vi "MoveSinglePIMotor.vi"(0 "System no.":i32=1 min=1 step=1, 1 "Axes to move":string[](array[string]), 2 "Move":dbl[](array[numeric]) format="%.6f", 3 "SafeMax":dbl[](array[numeric]) format="%.6f", 4 "SafeMin":dbl[](array[numeric]) format="%.6f", 5 "error in":errorcluster, 6 "Define home":bool, 7 "Move relative (-)":bool, 8 "Go home":bool, 9 "Move relative (+)":bool, 11 "Move absolute":bool, 12 "Stop refnum":refnum<vi>) -> (15 "Position":dbl[](array[numeric]) format="%.6f", 19 "error out":errorcluster)   [LabVIEW 2013]
doc: "This VI is runs in a loop until the stop button is pressed, the stop reference is TRUE or an error occures. It lets the operator set the velocity, move the connected axes to relative, absolute or to the home position, and reads the current position continuosly. The diagram shows how to combine the driver and support VIs for these tasks. Use the Help?Show Context Help menu sequence in the LabVIEW environment to display the Context Help window with the VI and control/indicator descriptions.\nRun \" XXXX_Configuration_Setup.vi\" (with XXXX being the PI product number of your system) prior to running this VI. \n\nValid for: C-843, C-843.PM, C-865, C-866, Mercury"
uses:
  C:/Users/Public/PI/GCSMergedLabVIEW/Low Level/General command.llb/Global2 (Array).vi
panel:
  in  "Clear":bool
  in  "stop":bool
  out "Conn. Axes":string[](array[string])
  # "Command move:"
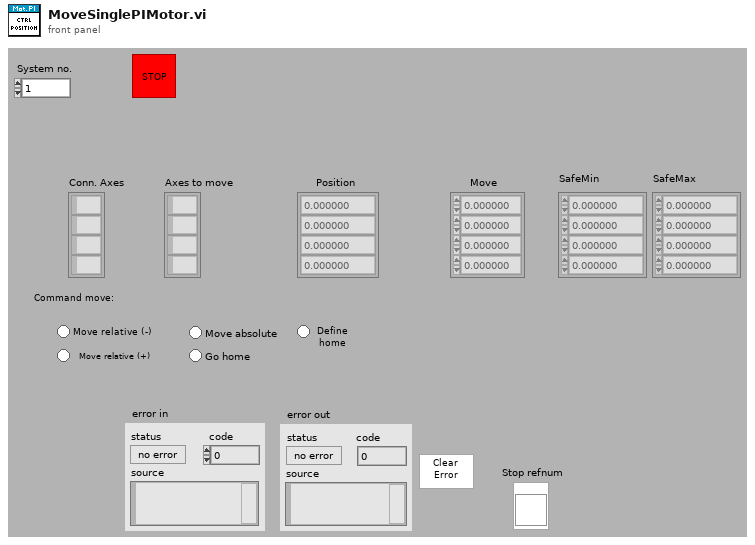
[diagram p1: front panel]
types:
  T1 = typedef "Controller names.ctl" = enum16{"None", "Analog", "C-702", "C-413", "C-843", "C-843.PM", "C-844", "C-848", "C-865", "C-866", "C-867", "C-877", "C-880", "C-884", "C-885", "C-891", "E-516", "E-517", "E-518", "E-709", "E-710", "E-712", "E-725", "E-727", "E-753", "E-754", "E-755", "E-761", "E-816", "E-861", "E-870", "E-871", "E-873", "F-206", "HydraPollux", "M-840", "M-850", "M-8X0", "Mercury", "Mercury_GCS"}
  T2 = cluster{"Conn. axes":string[], "Controller name":T1}[]
  T3 = cluster{"Conn. axes":string[], "Controller name":T1}
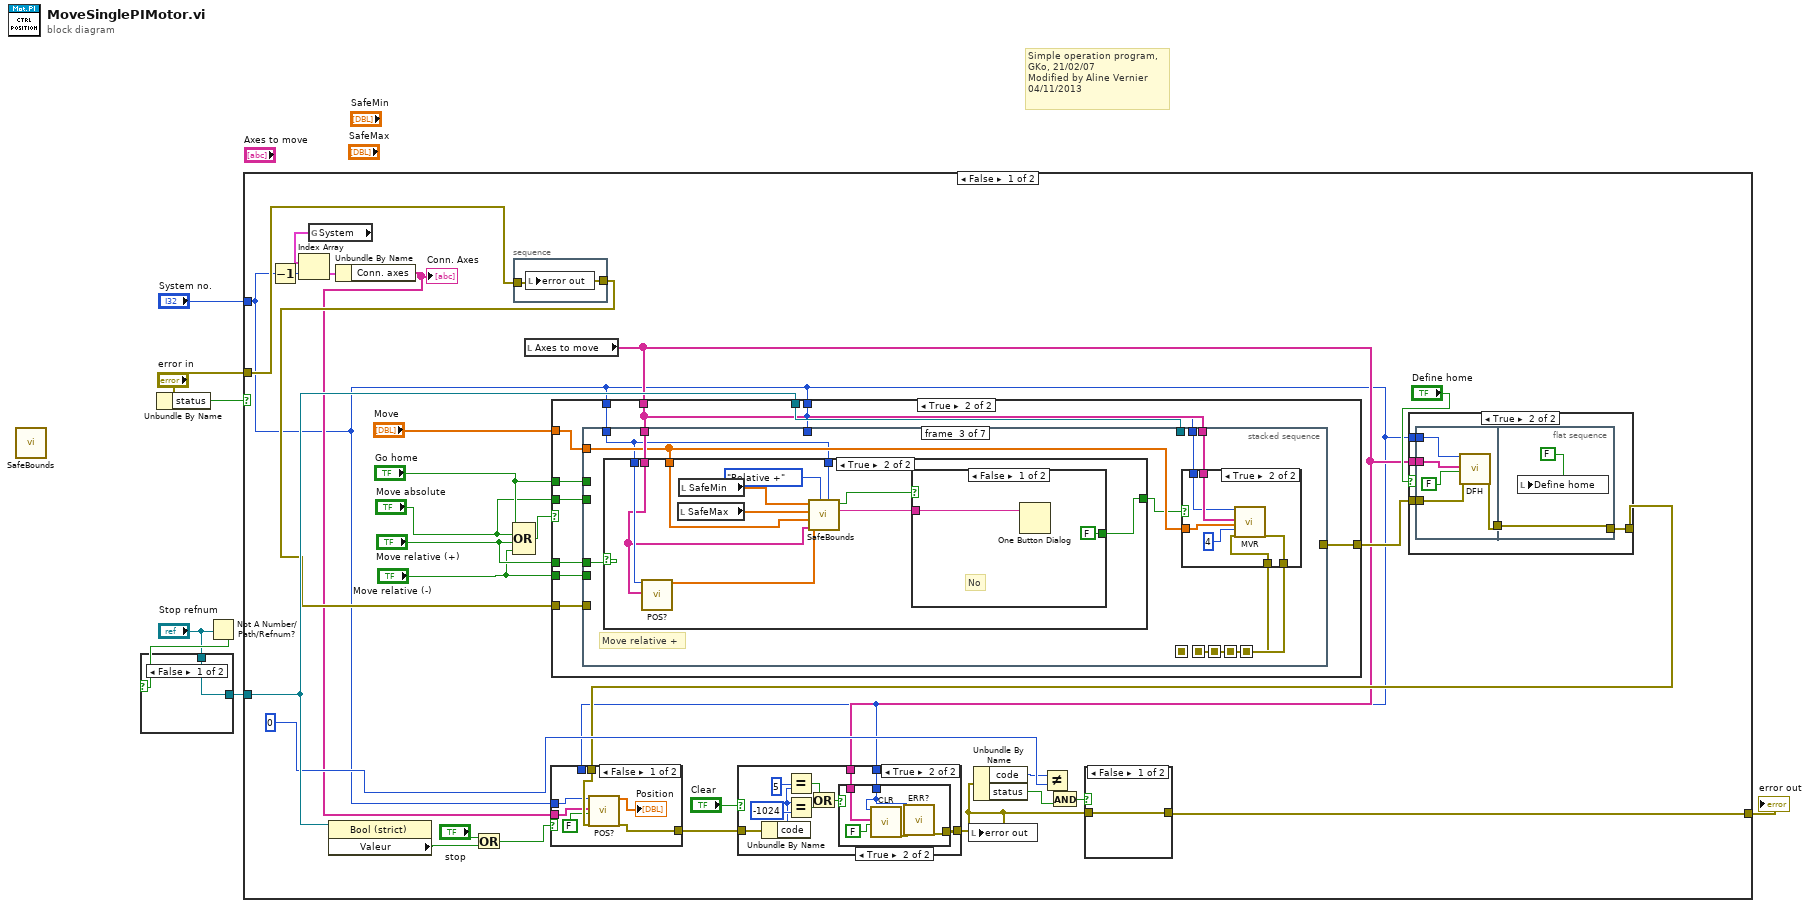
[diagram p0: block diagram]
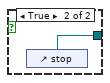
[diagram p2: hidden frame]
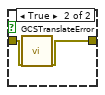
[diagram p3: hidden frame]
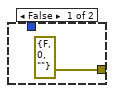
[diagram p5: hidden frame]
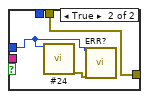
[diagram p6: hidden frame]
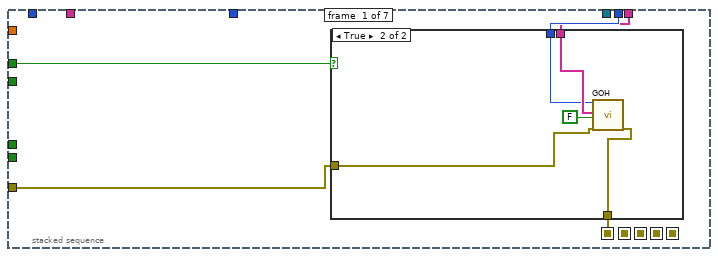
[diagram p8: hidden frame]
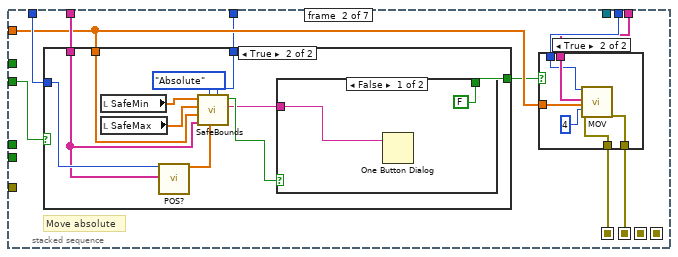
[diagram p10: hidden frame]
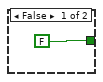
[diagram p11: hidden frame]
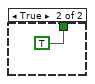
[diagram p12: hidden frame]
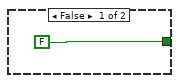
[diagram p14: hidden frame]
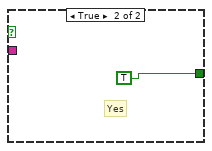
[diagram p15: hidden frame]
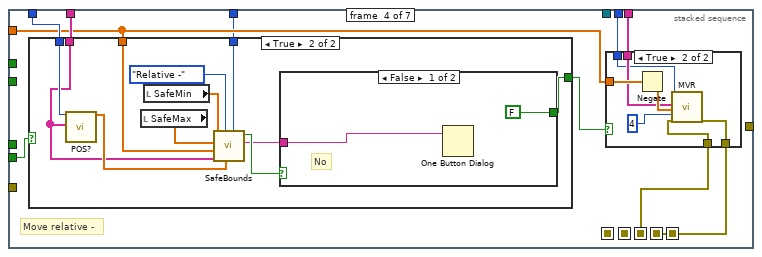
[diagram p17: hidden frame]
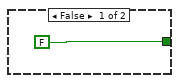
[diagram p18: hidden frame]
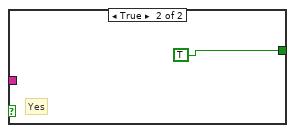
[diagram p19: hidden frame]
diagram:
  # "Simple operation program,\nGKo, 21/02/07\nModified by Aline Vernier\n04/11/2013"
  n1 = call "SafeBounds.vi"() -> ()  [unwired: 9 in, 3 out]
  n2 = Unbundle By Name("error in") -> ("status"=w6:bool)
  n3 = Not A Number/Path/Refnum?(number/path/refnum="Stop refnum") -> (NaN/Path/Refnum?=w3:bool)
  n4 = case shown="False" w3 {
    tunnel: [w8 w9] -> w2
    tunnel: "Stop refnum" -> [w8 _]
    frame False {
    }
    frame True {
      n5 = control-ref of="stop"() -> (w9:refnum<vi>)
    }
  }
  n6 = case shown="False" w6 {
    tunnel: [w39 w220] -> w5
    tunnel: "error in" -> [w38 w220]
    tunnel: "System no." -> [w10 _]
    tunnel: w2 -> [w37 _]
    frame False {
      n7 = Decrement(x=w10) -> (x-1=w35:i32)
      n8 = global read "Global2 (Array).vi" "System"() -> (w34:T2)
      n9 = Index Array(array=w34, index=w35) -> (element=w33:T3)
      n10 = property class="Bool (strict)"(reference=w37) -> ("Valeur"=w27:bool)  [unwired: 1 in, 2 out]
      n11 = Unbundle By Name(w33) -> ("Conn. axes"=w12:string[])
      "Conn. Axes" <- w12
      n12 = Or(x="stop", y=w27) -> (x .or. y?=w13:bool)
      n13 = Compound Arithmetic op=OR("Go home", "Move absolute", "Move relative (+)", "Move relative (-)") -> (w15:bool)
      n14 = stacked-sequence {
        tunnel: w38 -> [w219]
        tunnel: [w219] -> w32
        frame #0 {
          n15 = local write "error out"(w219) -> ()
        }
      }
      n16 = local read "Axes to move"() -> (w14:string[])
      n17 = case shown="True" w15 {
        tunnel: "Go home" -> [_ w80]
        tunnel: w10 -> [_ w70]
        tunnel: w14 -> [_ w71]
        tunnel: "Move" -> [_ w79]
        tunnel: [w69 w78] -> w26
        tunnel: w37 -> [_ w77]
        tunnel: "Move absolute" -> [_ w76]
        tunnel: "Move relative (+)" -> [_ w75]
        tunnel: w32 -> [w69 w74]
        tunnel: "Move relative (-)" -> [_ w73]
        tunnel: w10 -> [_ w72]
        frame False {
        }
        frame True {
          n18 = stacked-sequence {
            seq-local: [w82 _ _ _ _ _ _] -> [_ w99 _ _ _ _ _]
            seq-local: [_ w98 _ _ _ _ _] -> [_ _ w129 _ _ _ _]
            seq-local: [_ _ w130 _ _ _ _] -> [_ _ _ w162 _ _ _]
            seq-local: [_ _ _ w161 _ _ _] -> [_ _ _ _ w194 _ _]
            seq-local: [_ _ _ _ w193 _ _] -> [_ _ _ _ _ _ w198]
            tunnel: w80 -> [w85 _ _ _ _ _ _]
            tunnel: w70 -> [w84 w101 w132 w164 w189 _ w199]
            tunnel: w71 -> [w83 w100 w131 w163 w190 _ _]
            tunnel: w79 -> [_ w94 w126 w157 _ _ _]
            tunnel: [_ _ _ _ _ _ w200] -> w78
            tunnel: w77 -> [_ _ _ _ w188 _ _]
            tunnel: w76 -> [_ w97 _ _ _ _ _]
            tunnel: w75 -> [_ _ w128 _ _ _ _]
            tunnel: w74 -> [w81 _ _ _ _ _ _]
            tunnel: w73 -> [_ _ _ w160 _ _ _]
            tunnel: w72 -> [_ w96 w124 w159 _ _ _]
            tunnel: w71 -> [_ w95 w127 w158 _ _ _]
            tunnel: w70 -> [_ w92 _ w155 _ _ _]
            frame #0 {
              n19 = case shown="True" w85 {
                tunnel: w84 -> [_ w87]
                tunnel: w83 -> [_ w91]
                tunnel: [w86 w88] -> w82
                tunnel: w81 -> [w86 w89]
                frame False {
                }
                frame True {
                  n20 = call "GOH.vi"("System no."=w87, "GOH axes"=w91, "All axes?"=FALSE, "error in"=w89) -> ("error out"=w88:errorcluster)  [unwired: 15 in]
                }
              }
            }
            frame #1 {
              # "Move absolute"
              n21 = case shown="True" w97 {
                tunnel: w96 -> [_ w106]
                tunnel: w95 -> [_ w105]
                tunnel: w94 -> [_ w109]
                tunnel: [FALSE w113] -> w93
                tunnel: w92 -> [_ w103]
                frame False {
                }
                frame True {
                  n22 = local read "SafeMin"() -> (w111:dbl[])
                  n23 = local read "SafeMax"() -> (w110:dbl[])
                  n24 = call "POS?.vi"("System no."=w106, "Axes to query"=w105) -> ("Position"=w104:dbl[])  [unwired: 16 in, 1 out]
                  n25 = call "SafeBounds.vi"("System no."=w103, "Position"=w104, "Type of movement"=enum16{"Relative -", "Relative +", "Absolute"}."Absolute", "Axes to move"=w105, "Move"=w109, "SafeMax"=w110, "SafeMin"=w111) -> ("Message"=w107:string, "All good?"=w108:bool)  [unwired: 2 in, 1 out]
                  n26 = case shown="False" w108 {
                    tunnel: [FALSE TRUE] -> w113
                    tunnel: w107 -> [w114 _]
                    frame False {
                      n27 = One Button Dialog(message=w114) -> ()  [unwired: 1 in, 1 out]
                    }
                    frame True {
                    }
                  }
                }
              }
              n28 = case shown="True" w93 {
                tunnel: w101 -> [_ w120]
                tunnel: w100 -> [_ w121]
                tunnel: w99 -> [w117 w122]
                tunnel: w94 -> [_ w118]
                tunnel: [w117 w119] -> w98
                frame False {
                }
                frame True {
                  n29 = call "MOV.vi"("System no."=w120, "Axes to move"=w121, "Position values"=w118, "No.of digits"=i16 4, "error in"=w122) -> ("error out"=w119:errorcluster)  [unwired: 14 in]
                }
              }
            }
            frame #2 {
              # "Move relative +"
              n30 = case shown="True" w128 {
                tunnel: [FALSE w143] -> w125
                tunnel: w124 -> [_ w144]
                tunnel: w127 -> [_ w138]
                tunnel: w126 -> [_ w139]
                tunnel: w124 -> [_ w136]
                frame False {
                }
                frame True {
                  n31 = call "POS?.vi"("System no."=w144, "Axes to query"=w138) -> ("Position"=w137:dbl[])  [unwired: 16 in, 1 out]
                  n32 = local read "SafeMax"() -> (w140:dbl[])
                  n33 = local read "SafeMin"() -> (w141:dbl[])
                  n34 = call "SafeBounds.vi"("System no."=w136, "Position"=w137, "Type of movement"=enum16{"Relative -", "Relative +", "Absolute"}."Relative +", "Axes to move"=w138, "Move"=w139, "SafeMax"=w140, "SafeMin"=w141) -> ("Message"=w134:string, "All good?"=w135:bool)  [unwired: 2 in, 1 out]
                  n35 = case shown="False" w135 {
                    tunnel: [FALSE TRUE] -> w143
                    tunnel: w134 -> [w145 _]
                    frame False {
                      # "No"
                      n36 = One Button Dialog(message=w145) -> ()  [unwired: 1 in, 1 out]
                    }
                    frame True {
                      # "Yes"
                    }
                  }
                }
              }
              n37 = case shown="True" w125 {
                tunnel: w132 -> [_ w151]
                tunnel: w131 -> [_ w152]
                tunnel: w126 -> [_ w153]
                tunnel: [w148 w149] -> w130
                tunnel: w129 -> [w148 w150]
                frame False {
                }
                frame True {
                  n38 = call "MVR.vi"("System no."=w151, "Axes to move"=w152, "Position values"=w153, "No.of digits"=i16 4, "error in"=w150) -> ("error out"=w149:errorcluster)  [unwired: 14 in]
                }
              }
            }
            frame #3 {
              # "Move relative -"
              n39 = case shown="True" w160 {
                tunnel: [FALSE w174] -> w156
                tunnel: w159 -> [_ w175]
                tunnel: w158 -> [_ w171]
                tunnel: w157 -> [_ w173]
                tunnel: w155 -> [_ w167]
                frame False {
                }
                frame True {
                  n40 = call "POS?.vi"("System no."=w175, "Axes to query"=w171) -> ("Position"=w172:dbl[])  [unwired: 16 in, 1 out]
                  n41 = local read "SafeMax"() -> (w169:dbl[])
                  n42 = local read "SafeMin"() -> (w170:dbl[])
                  n43 = call "SafeBounds.vi"("System no."=w167, "Position"=w172, "Type of movement"=enum16{"Relative -", "Relative +", "Absolute"}."Relative -", "Axes to move"=w171, "Move"=w173, "SafeMax"=w169, "SafeMin"=w170) -> ("Message"=w166:string, "All good?"=w176:bool)  [unwired: 2 in, 1 out]
                  n44 = case shown="False" w176 {
                    tunnel: [FALSE TRUE] -> w174
                    tunnel: w166 -> [w177 _]
                    frame False {
                      # "No"
                      n45 = One Button Dialog(message=w177) -> ()  [unwired: 1 in, 1 out]
                    }
                    frame True {
                      # "Yes"
                    }
                  }
                }
              }
              n46 = case shown="True" w156 {
                tunnel: w164 -> [_ w183]
                tunnel: w163 -> [_ w184]
                tunnel: w157 -> [_ w187]
                tunnel: w162 -> [w180 w182]
                tunnel: [w180 w181] -> w161
                frame False {
                }
                frame True {
                  n47 = Negate(x=w187) -> (-x=w185:dbl[])
                  n48 = call "MVR.vi"("System no."=w183, "Axes to move"=w184, "Position values"=w185, "No.of digits"=i16 4, "error in"=w182) -> ("error out"=w181:errorcluster)  [unwired: 14 in]
                }
              }
            }
            frame #4 {
              n49 = call "Wait for axes to stop.vi"("System no."=w189, "Axes to wait for"=w190, "With status bit polling?"=FALSE, "error in"=w194, "Polling cycle time, ms"=u32 50, "Stop refnum"=w188) -> ("error out"=w193:errorcluster)  [unwired: 12 in, 1 out]
            }
            frame #5 {
              w195 = FALSE ("Go home")
              n50 = local write "Move absolute"(w195) -> ()
              n51 = local write "Go home"(w195) -> ()
              n52 = local write "Move relative (+)"(w195) -> ()
              n53 = local write "Move relative (-)"(w195) -> ()
            }
            frame #6 {
              n54 = call "ERR?.vi"("System no."=w199, "error in"=w198) -> ("error out"=w197:errorcluster)  [unwired: 16 in, 1 out]
              n55 = Unbundle By Name(w197) -> ("code"=w196:i32)
              n56 = Equal?(x=7 ("y"), y=w196) -> (x = y?=w201:bool)
              n57 = case shown="False" w201 {
                tunnel: [w203 w204] -> w200
                tunnel: w198 -> [_ w204]
                tunnel: w197 -> [w203 _]
                frame False {
                }
                frame True {
                  n58 = One Button Dialog(message="Position out of range") -> ()  [unwired: 1 in, 1 out]
                }
              }
            }
          }
        }
      }
      n59 = case shown="True" "Define home" {
        tunnel: w10 -> [_ w211]
        tunnel: w14 -> [_ w210]
        tunnel: w26 -> [w206 w209]
        tunnel: [w206 w208] -> w25
        frame False {
        }
        frame True {
          n60 = flat-sequence {
            tunnel: w211 -> [w216]
            tunnel: w210 -> [w215]
            tunnel: w209 -> [w213]
            tunnel: [w212] -> w207
            tunnel: [w218] -> w208
            tunnel: w207 -> [w218]
            frame #0 {
              n61 = call "DFH.vi"("System no."=w216, "DFH axes"=w215, "All axes?"=FALSE, "error in"=w213) -> ("error out"=w212:errorcluster)  [unwired: 15 in]
            }
            frame #1 {
              n62 = local write "Define home"(FALSE ("All axes?")) -> ()
            }
          }
        }
      }
      n63 = case shown="False" w13 {
        tunnel: w10 -> [w60 w67]
        tunnel: w10 -> [_ _]
        tunnel: w25 -> [w63 w68]
        tunnel: [w64 w68] -> w23
        tunnel: w12 -> [w61 _]
        frame False {
          n64 = call "POS?.vi"("System no."=w60, "Axes to query"=w61, "All axes?"=FALSE, "error in"=w63) -> ("Position"=→"Position":dbl[], "error out"=w64:errorcluster)  [unwired: 14 in]
        }
        frame True {
          n65 = call "#24.vi"("System no."=w67) -> ("error out"=w66:errorcluster)  [unwired: 18 in]
          n66 = call "ERR?.vi"("System no."=w67, "error in"=w66) -> ()  [unwired: 16 in, 2 out]
        }
      }
      n67 = case shown="True" "Clear" {
        tunnel: [w43 w46] -> w19
        tunnel: w23 -> [w43 w50]
        tunnel: w10 -> [_ w45]
        tunnel: w14 -> [_ w44]
        frame False {
        }
        frame True {
          n68 = Unbundle By Name(w50) -> ("code"=w51:i32)
          n69 = Equal?(x=5 ("y"), y=w51) -> (x = y?=w49:bool)
          n70 = Equal?(x=w51, y=-1024) -> (x = y?=w47:bool)
          n71 = Or(x=w49, y=w47) -> (x .or. y?=w48:bool)
          n72 = case shown="True" w48 {
            tunnel: [errorcluster {"status"=FALSE, "code"=0, "source"=""} ("error out") w55] -> w46
            tunnel: w45 -> [_ w58]
            tunnel: w44 -> [_ w57]
            frame False {
            }
            frame True {
              n73 = call "CLR.vi"("System no."=w58, "CLR axes"=w57, "All axes?"=FALSE) -> ("error out"=w59:errorcluster)  [unwired: 16 in]
              n74 = call "ERR?.vi"("System no."=w58, "error in"=w59) -> ("error out"=w55:errorcluster)  [unwired: 16 in, 1 out]
            }
          }
        }
      }
      n75 = local write "error out"(w19) -> ()
      n76 = Unbundle By Name(w19) -> ("code"=w22:i32, "status"=w18:bool)
      n77 = Not Equal?(x=w22, y=0 ("code")) -> (x != y?=w21:bool)
      n78 = And(x=w21, y=w18) -> (x .and. y?=w20:bool)
      n79 = case shown="False" w20 {
        tunnel: w19 -> [w40 w42]
        tunnel: [w40 w41] -> w39
        frame False {
        }
        frame True {
          n80 = call "GCSTranslateError.vi"("error in"=w42) -> ("error out"=w41:errorcluster)  [unwired: 16 in, 2 out]
        }
      }
    }
    frame True {
      (unwired) FALSE ("stop")
    }
  }
  "error out" <- w5
